vi "Open-Close ALL Relays.vi"(8 "error in (no error)":errorcluster, 9 "Ignored Relays (empty)":string[](array[string]), 10 "State":bool, 11 "DAQ in":refnum<class "DAQ.lvclass">) -> (0 "error out":errorcluster, 3 "DAQ out":refnum<class "DAQ.lvclass">)   [LabVIEW 2017, in "DAQ.lvclass"]
doc: "Developed by Kevin Thompson\nkevin@thompsonengineering.net\n\nCopyright 2015\nThompson Engineering, LLC"
uses:
  DAQ.lvclass
  DAQ.lvclass/DAQ.ctl
  Accessors/Get DAQ Settings.vi
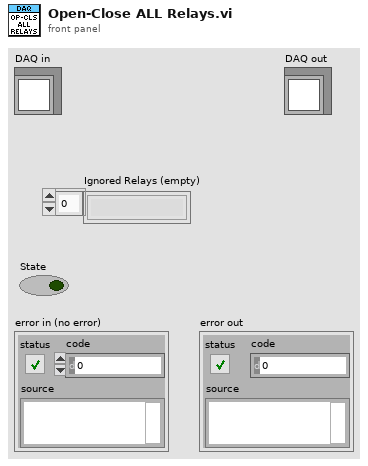
[diagram p1: front panel]
types:
  T1 = typedef "DAQ.lvclass/TD DAQ Settings--cluster.ctl" = cluster{"Simulate DAQ":bool, "DI Settings":T2[], "AI Settings":T3[], "Relay IONames":string[], "AO IONames":string[], "AO NChan SingleTask":bool}
  T2 = typedef "DAQ.lvclass/TD DI Instrument Settings--cluster.ctl" = cluster{"Disable":bool, "DI TaskName":string, "DI RefreshIntv":i32}
  T3 = typedef "DAQ.lvclass/TD AI Instrument Settings--cluster.ctl" = cluster{"Disable":bool, "AI TaskName":string, "AI InstSettings":T4, "SimAI Ranges":T5}
  T4 = typedef "DAQ.lvclass/TD AI InstSettings--cluster.ctl" = cluster{"DaqRate":dbl, "NumSamples":i32}
  T5 = typedef "DAQ.lvclass/TD SimAI Ranges--cluster.ctl" = cluster{"lo":dbl, "hi":dbl}
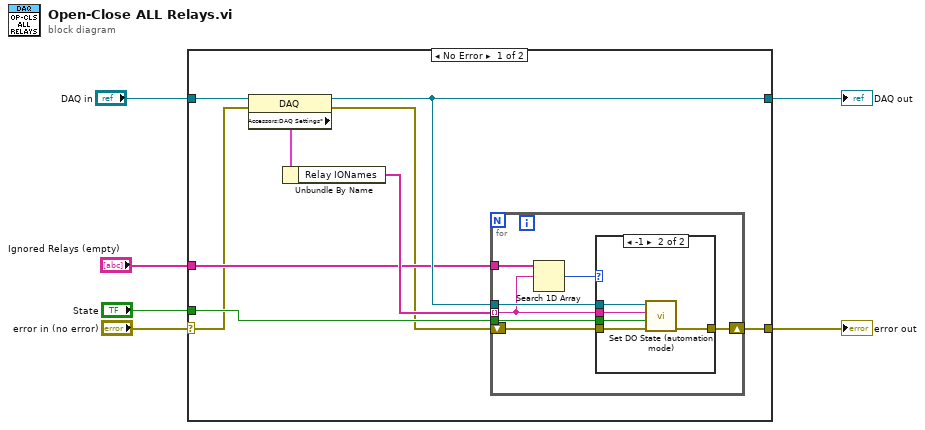
[diagram p0: block diagram]
diagram:
  n1 = case shown="No Error" "error in (no error)" {
    selector: "error in (no error)" -> [w8 w30]
    tunnel: [w15 w30] -> w6
    tunnel: "State" -> [w14 _]
    tunnel: "DAQ in" -> [w12 w29]
    tunnel: [w11 w29] -> w3
    tunnel: "Ignored Relays (empty)" -> [w9 _]
    frame No Error {
      n2 = property class="DAQ"(reference=w12, error in=w8) -> (reference out=w11:refnum<class "DAQ.lvclass">, error out=w7:errorcluster, "Accessors:DAQ Settings*"=w13:T1)
      n3 = Unbundle By Name(w13) -> ("Relay IONames"=w10:string[])
      n4 = for {
        tunnel: w11 -> [w22]
        tunnel: w14 -> [w21]
        shift-right: [w19] -> w15
        shift-left: w7 -> [w20]
        tunnel: w10 -> [w17] mode=indexing
        tunnel: w9 -> [w18]
        n5 = Search 1D Array(1D array=w18, element=w17) -> (index of element=w16:i32)  [unwired: 1 in]
        n6 = case shown="-1" w16 {
          tunnel: w22 -> [_ w28]
          tunnel: w21 -> [_ w27]
          tunnel: w20 -> [w23 w26]
          tunnel: [w23 w25] -> w19
          tunnel: w17 -> [_ w24]
          frame 0, Default {
          }
          frame -1 {
            n7 = call "Set DO State (automation mode).vi"("error in (no error)"=w26, "State"=w27, "DO IOName"=w24, "DAQ"=w28) -> ("error out"=w25:errorcluster)  [unwired: 6 in, 1 out]
          }
        }
      }
    }
    frame Error {
    }
  }
  "error out" <- w6
  "DAQ out" <- w3
